vi "Integral_tests.vi"() -> ()   [LabVIEW 2013]
uses:
  <vilib>/Analysis/NI_AALPro.lvlib
  <vilib>/Analysis/8numeric.llb/1D Numeric Integration.vi
panel:
  out "Delta E3":dbl
  out "Delta E2":dbl
  out "Delta E":dbl
  out "Real function":dbl
  out "Array 2":dbl[](array[numeric])
  out "Array":dbl[](array[numeric])
  out "dx":dbl
  out "XY Graph":cluster{dbl[], "Integral X":dbl[]}[](graph)
  out "Integral definida":dbl
  out "My integral":dbl
  in  "Number of iterations":i32
  out "Numeric integral":dbl format="%0.4f"
  in  "Max":i32
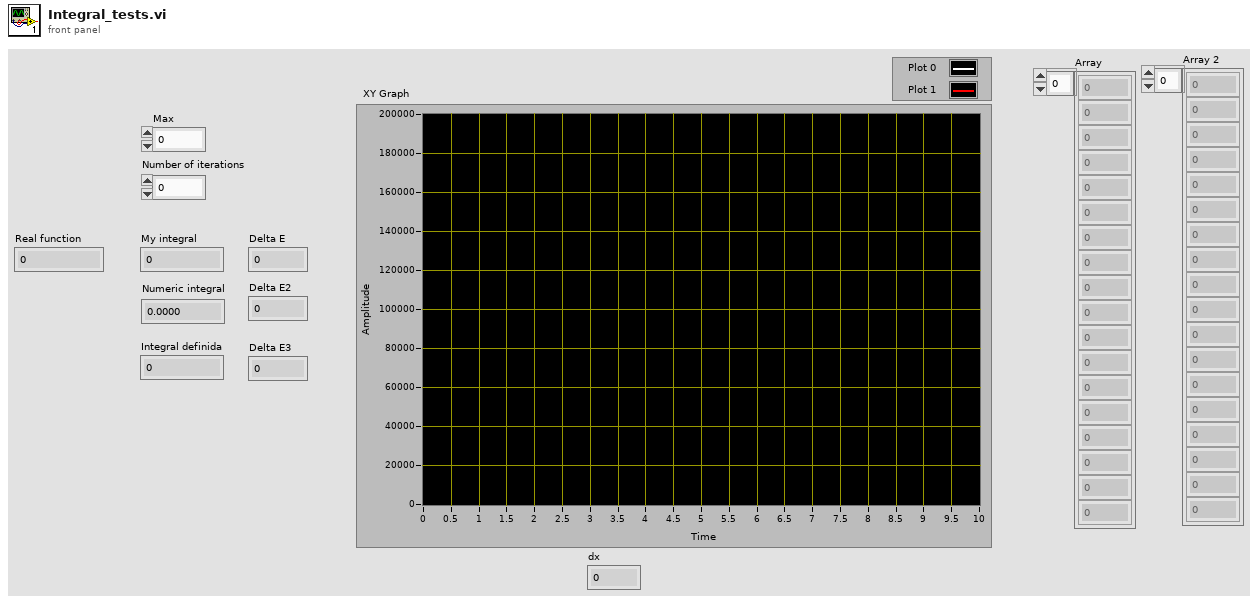
[diagram p1: front panel]
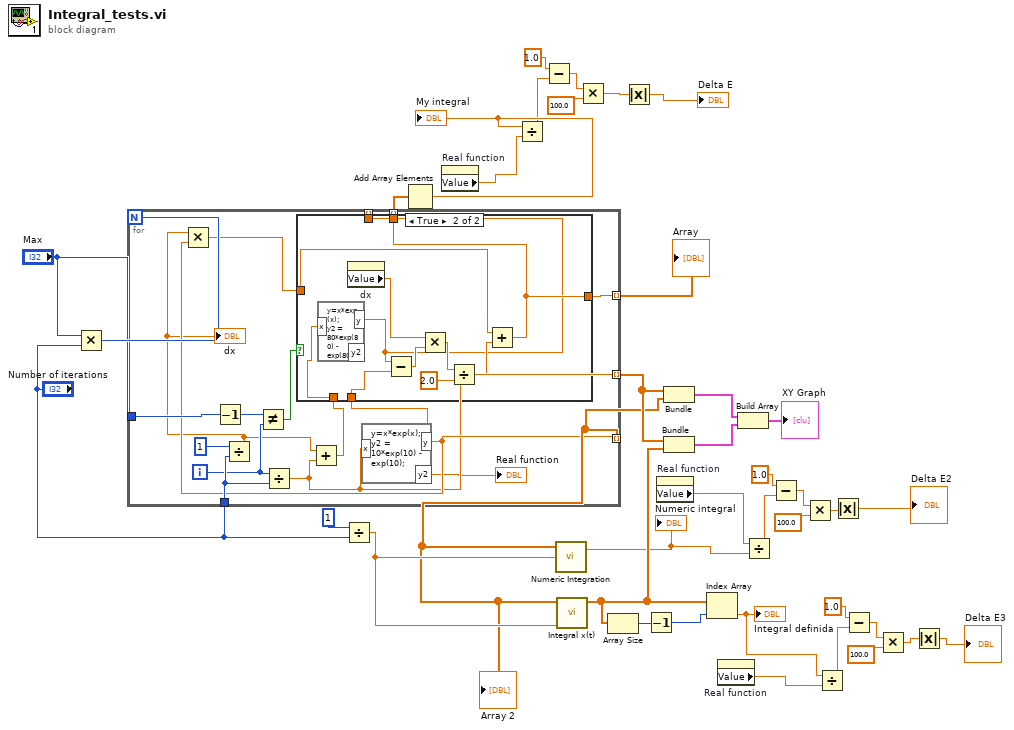
[diagram p0: block diagram]
diagram:
  n1 = Multiply(x="Max", y="Number of iterations") -> (x*y=w39:i32)
  n2 = for {
    N: w39 -> [_]
    tunnel: [w47] -> w28 mode=indexing
    tunnel: "Number of iterations" -> [w53]
    tunnel: [w44] -> w29 mode=indexing
    tunnel: "Max" -> [w52]
    tunnel: [w48] -> w27 mode=indexing
    tunnel: [w46] -> w25 mode=indexing
    tunnel: [w45] -> _ mode=indexing
    i -> [w50]
    n3 = Decrement(x=w52) -> (x-1=w51:i32)
    n4 = Divide(x=1, y=w53) -> (x/y=w43:dbl)
    "dx" <- w43
    n5 = Not Equal?(x=w51, y=w50) -> (x != y?=w40:bool)
    n6 = Divide(x=w50, y=w53) -> (x/y=w44:dbl)
    n7 = Add(x=w43, y=w44) -> (x+y=w42:dbl)
    n8 = formula code="y=x*exp(x);\ny2 = 10*exp(10) - exp(10);"("x"=w44) -> ("y"=w47:dbl, "y2"=→"Real function":dbl)
    n9 = Multiply(x=w43, y=w47) -> (x*y=w49:dbl)
    n10 = case shown="True" w40 {
      tunnel: w49 -> [w55 w59]
      tunnel: w47 -> [_ w62]
      tunnel: w42 -> [_ w56]
      tunnel: [w55 w58] -> w48
      tunnel: [w55 w58] -> w46
      tunnel: [w55 w57] -> w45
      frame False {
      }
      frame True {
        n11 = formula code="y=x*exp(x);\ny2 = 80*exp(80) - exp(80);"("x"=w56) -> ("y"=w57:dbl)  [unwired: 1 out]
        n12 = property on="dx" class="DigNum (strict)"() -> ("Value"=w61:dbl)  [unwired: 2 in, 2 out]
        n13 = Subtract(x=w57, y=w62) -> (x-y=w65:dbl)
        n14 = Multiply(x=w61, y=w65) -> (x*y=w64:dbl)
        n15 = Divide(x=w64, y=2.0) -> (x/y=w60:dbl)
        n16 = Add(x=w59, y=w60) -> (x+y=w58:dbl)
      }
    }
  }
  "Array" <- w25
  "Array 2" <- w28
  n17 = Divide(x=1, y="Number of iterations") -> (x/y=w36:dbl)
  n18 = Add Array Elements(numeric array=w27) -> (sum=w20:dbl)
  "My integral" <- w20
  n19 = property on="Real function" class="DigNum (strict)"() -> ("Value"=w21:dbl)  [unwired: 2 in, 2 out]
  n20 = Divide(x=w20, y=w21) -> (x/y=w19:dbl)
  n21 = Subtract(x=1.0 ("x/y"), y=w19) -> (x-y=w23:dbl)
  n22 = call-poly <vilib>:"Numeric Integration.vi"("dt"=w36, "Input Array"=w28) -> ("result"=w13:dbl)  [unwired: 1 in, 1 out]
  "Numeric integral" <- w13
  n23 = call <vilib>:"Integral x(t).vi"("dt"=w36, "X"=w28) -> ("Integral X"=w33:dbl[])  [unwired: 8 in, 1 out]
  n24 = Multiply(x=w23, y=100.0) -> (x*y=w2:dbl)
  n25 = Array Size(array=w33) -> (size(s)=w38:i32)
  n26 = Absolute Value(x=w2) -> (abs(x)=→"Delta E":dbl)
  n27 = Decrement(x=w38) -> (x-1=w37:i32)
  n28 = property on="Real function" class="DigNum (strict)"() -> ("Value"=w14:dbl)  [unwired: 2 in, 2 out]
  n29 = Bundle(w29, w28) -> (w32:cluster{dbl[], dbl[]})  [unwired: 1 in]
  n30 = Bundle(w29, "Integral X"=w33) -> (w31:cluster{dbl[], "Integral X":dbl[]})  [unwired: 1 in]
  n31 = Index Array(array=w33, index=w37) -> (element=w8:dbl)
  "Integral definida" <- w8
  n32 = property on="Real function" class="DigNum (strict)"() -> ("Value"=w7:dbl)  [unwired: 2 in, 2 out]
  n33 = Build Array(w32, w31) -> (→"XY Graph":cluster{dbl[], "Integral X":dbl[]}[])
  n34 = Divide(x=w14, y=w13) -> (x/y=w15:dbl)
  n35 = Subtract(x=1.0 ("x/y"), y=w15) -> (x-y=w17:dbl)
  n36 = Multiply(x=w17, y=100.0) -> (x*y=w6:dbl)
  n37 = Divide(x=w8, y=w7) -> (x/y=w9:dbl)
  n38 = Absolute Value(x=w6) -> (abs(x)=→"Delta E2":dbl)
  n39 = Subtract(x=1.0 ("x/y"), y=w9) -> (x-y=w11:dbl)
  n40 = Multiply(x=w11, y=100.0) -> (x*y=w4:dbl)
  n41 = Absolute Value(x=w4) -> (abs(x)=→"Delta E3":dbl)
